vi "FFT - computation parameters.vi"(0 "Spectral Function Parameters":T2={"Frequency resolution (Hz)"=1.0, "Overlap"=0.0, "Window"=0} {"Window" items=["Rectangle"=0, "Hanning"=1, "Hamming"=2, "Blackman-Harris"=3, "Exact Blackman"=4, "Blackman"=5, "Flat Top"=6, "4 Term B-Harris "=7, "7 Term B-Harris"=8, "Low Sidelobe"=9, "Blackman Nuttall"=11, "Triangle"=30, "Bartlett-Hanning"=31, "Bohman"=32, "Parzen"=33, "Welch"=34, "Kaiser"=60, "Dolph-Chebyshev"=61, "Gaussian"=62]}, 4 "Fs":dbl, 5 "Time vector length (samples)":i32) -> (14 "Nb Averages":i32, 15 "FFT Length/2":i32, 16 "FFT Length - Overlap":i32, 17 "FFT Length":i32, 18 "Frequency resolution (Hz) OUT":dbl, 19 "window":T1 items=["Rectangle"=0, "Hanning"=1, "Hamming"=2, "Blackman-Harris"=3, "Exact Blackman"=4, "Blackman"=5, "Flat Top"=6, "4 Term B-Harris "=7, "7 Term B-Harris"=8, "Low Sidelobe"=9, "Blackman Nuttall"=11, "Triangle"=30, "Bartlett-Hanning"=31, "Bohman"=32, "Parzen"=33, "Welch"=34, "Kaiser"=60, "Dolph-Chebyshev"=61, "Gaussian"=62])   [LabVIEW 2022 SP3, in "GSwFormDSP.lvclass"]
uses:
  GSwFormDSP.lvclass
  Spectral Parameters.ctl
  <vilib>/Analysis/4window.llb/windowTd.ctl
  <vilib>/Analysis/NI_AALPro.lvlib
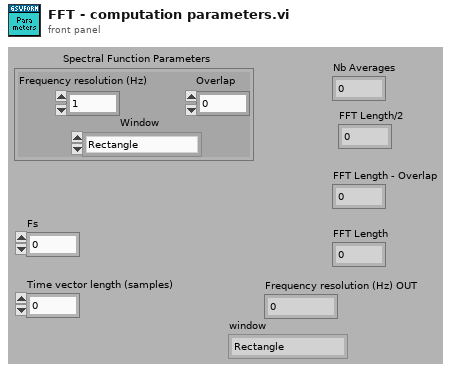
[diagram p1: front panel]
types:
  T1 = typedef "NI_AALPro.lvlib/windowTd.ctl" = u32
  T2 = typedef "GSwFormDSP.lvclass/Spectral Parameters.ctl" = cluster{"Frequency resolution (Hz)":dbl, "Overlap":dbl, "Window":T1}
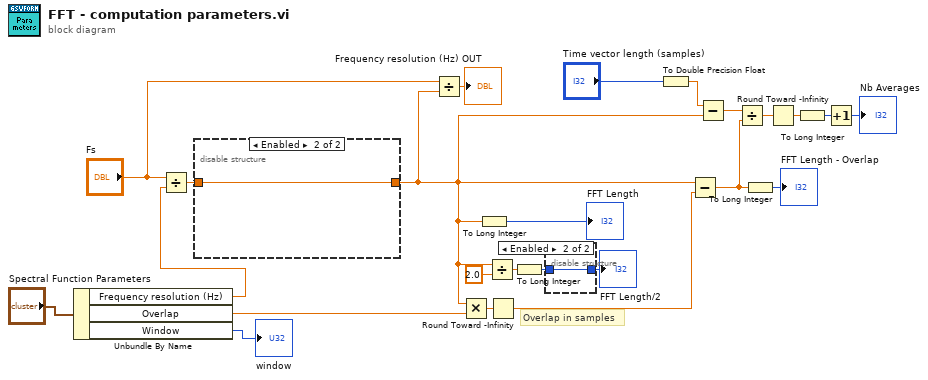
[diagram p0: block diagram]
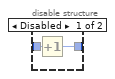
[diagram p2: hidden frame]
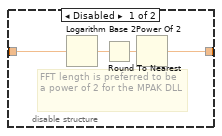
[diagram p3: hidden frame]
diagram:
  # "Overlap in samples"
  n1 = Unbundle By Name("Spectral Function Parameters") -> ("Frequency resolution (Hz)"=w8:dbl, "Overlap"=w7:dbl, "Window"=→"window":T1)
  n2 = Divide(x="Fs", y=w8) -> (x/y=w22:dbl)
  n3 = disable-structure shown="Enabled" {
    disable-tunnel: w22 -> [w26 w29]
    disable-tunnel: [w25 w29] -> w6
    frame Disabled {
      # "FFT length is preferred to be a power of 2 for the MPAK DLL"
      n4 = Logarithm Base 2(1:w26) -> (0:w28:dbl)
      n5 = Round To Nearest(number=w28) -> (nearest integer value=w27:dbl)
      n6 = Power Of 2(x=w27) -> (2^x=w25:dbl)
    }
    frame Enabled {
    }
  }
  n7 = Divide(x="Fs", y=w6) -> (x/y=→"Frequency resolution (Hz) OUT":dbl)
  n8 = Multiply(x=w6, y=w7) -> (x*y=w13:dbl)
  n9 = To Long Integer(number=w6) -> (32bit integer=→"FFT Length":i32)
  n10 = Divide(x=w6, y=2.0) -> (x/y=w4:dbl)
  n11 = Round Toward -Infinity(1:w13) -> (0:w18:dbl)
  n12 = To Long Integer(number=w4) -> (32bit integer=w3:i32)
  n13 = disable-structure shown="Enabled" {
    disable-tunnel: w3 -> [w31 w32]
    disable-tunnel: [w30 w32] -> w2
    frame Disabled {
      n14 = Increment(x=w31) -> (x+1=w30:i32)
    }
    frame Enabled {
    }
  }
  "FFT Length/2" <- w2
  n15 = To Double Precision Float(number="Time vector length (samples)") -> (double precision float=w16:dbl)
  n16 = Subtract(x=w6, y=w18) -> (x-y=w19:dbl)
  n17 = Subtract(x=w16, y=w6) -> (x-y=w17:dbl)
  n18 = Divide(x=w17, y=w19) -> (x/y=w12:dbl)
  n19 = To Long Integer(number=w19) -> (32bit integer=→"FFT Length - Overlap":i32)
  n20 = Round Toward -Infinity(1:w12) -> (0:w15:dbl)
  n21 = To Long Integer(number=w15) -> (32bit integer=w14:i32)
  n22 = Increment(x=w14) -> (x+1=→"Nb Averages":i32)
